vi "Start Function.vi"(8 "error in (no error)":errorcluster, 10 "Launch Functions Message in":refnum<class "Launch Functions Message.lvclass">, 11 "Controller in":refnum<class "Controller.lvclass">) -> (0 "error out":errorcluster, 3 "Controller out":refnum<class "Controller.lvclass">)   [LabVIEW 2016, in "Controller Actor.lvlib" / "Controller.lvclass"]
uses:
  <userlib>/Common Components/Controller/Controller.lvclass
  C:/Program Files (x86)/National Instruments/LabVIEW 2016/vi.lib/ActorFramework/Actor/Actor.lvclass
  <userlib>/Common Components/Controller/Messages/Launch Functions Message/Launch Functions Message.lvclass
  <userlib>/Common Components/Controller/Messages/Launch Functions Message/Launch Functions Message.lvclass/Launch Functions Message.ctl
  <userlib>/Common Components/Hardware/DevInfo/DevInfo.lvclass/DevInfo.ctl
  <userlib>/Common Components/Function Actor/Function.lvclass/Function.ctl
  <vilib>/ActorFramework/Actor/Actor.lvclass/Actor.ctl
  <vilib>/ActorFramework/Message Enqueuer/Message Enqueuer.lvclass/Message Enqueuer.ctl
  <userlib>/Common Components/Function Actor/Accessors/Write Time Function Requested.vi
  <userlib>/Common Components/Function Actor/Write GUID.vi
  <userlib>/Common Components/Function Actor/Accessors/Write Master_.vi
  <userlib>/Common Components/Function Actor/Accessors/Write WS Message Broker Interface Ref.vi
  <userlib>/Common Components/Function Actor/Accessors/Write HWplugin List LUT.vi
  <userlib>/Common Components/Controller/Messages/Launch Functions Message/Read Function Name.vi
  <userlib>/Common Components/Controller/Messages/Launch Functions Message/Read Devices.vi
  <userlib>/Common Components/Controller/Messages/Launch Functions Message/Read Show FP_.vi
  <userlib>/Common Components/Controller/Messages/Launch Functions Message/Read Time Function Requested 2.vi
  <userlib>/Common Components/Controller/Messages/Launch Functions Message/Read Master_.vi
  <vilib>/ActorFramework/Message Enqueuer/Init from Existing Queue.vi
  <userlib>/Common Components/Function Actor/Function.lvclass
  <userlib>/Common Components/Controller/Methods/Print List of Hardware (DevInfo).vi
  <userlib>/Common Components/Function Actor/Properties/Write Array of Hardware 2.vi
  <userlib>/Common Components/Function Actor/Properties/Write Show UI While Running 2.vi
  <userlib>/Common Components/Hardware/DevInfo/DevInfo.lvclass
  <userlib>/Common Components/Hardware/Abstract Hardware/Hardware.lvclass
  <vilib>/ActorFramework/Message Enqueuer/Message Enqueuer.lvclass
  <vilib>/ActorFramework/Actor/Actor.lvclass
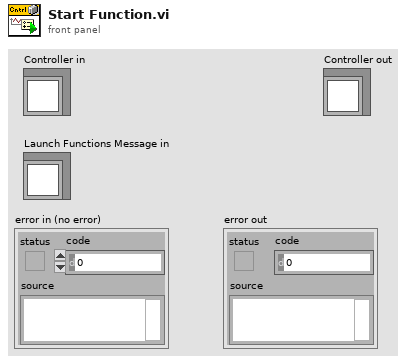
[diagram p1: front panel]
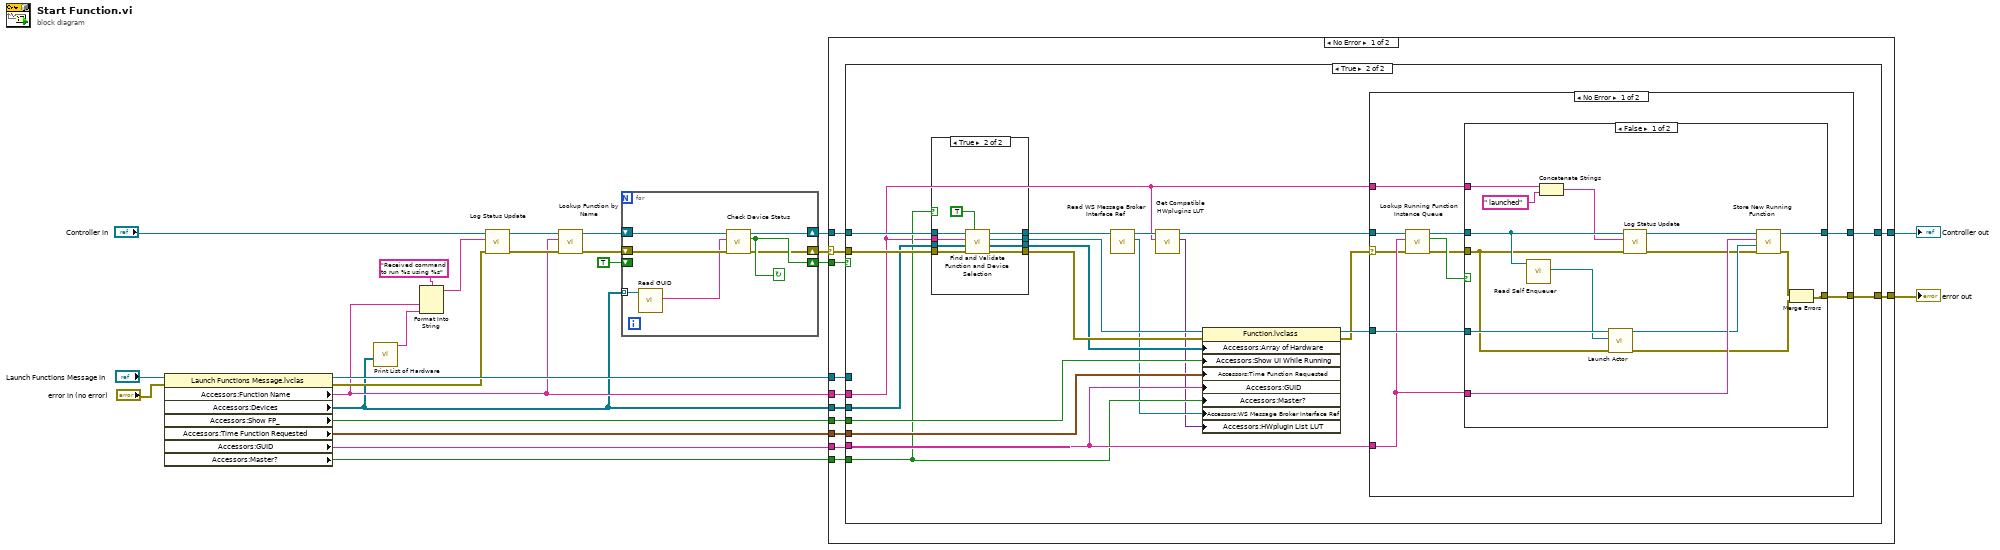
[diagram p0: block diagram]
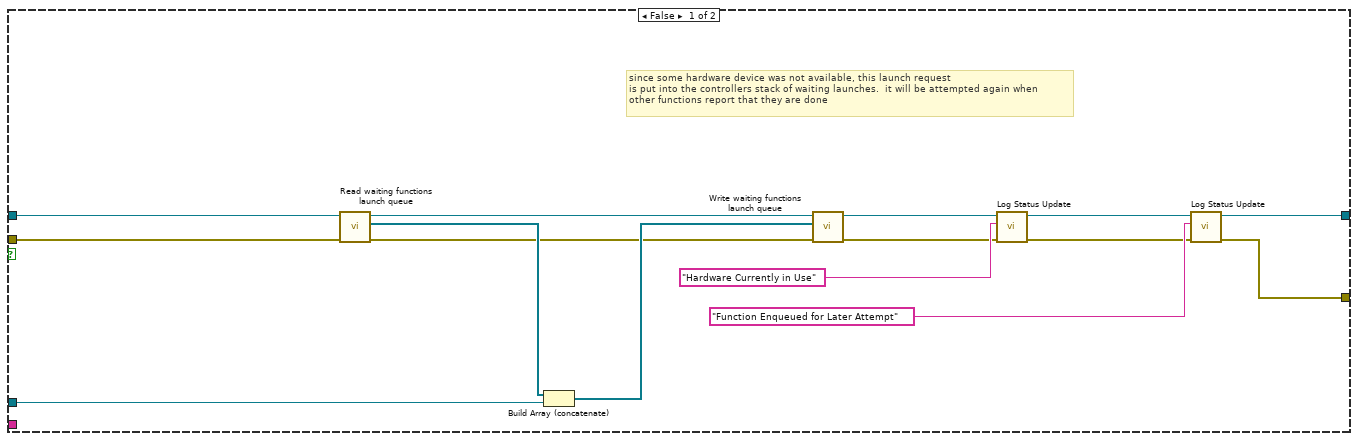
[diagram p2: hidden frame]
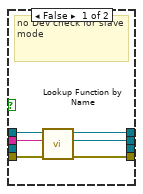
[diagram p3: hidden frame]
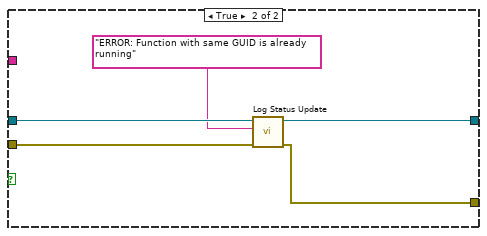
[diagram p4: hidden frame]
diagram:
  n1 = property class="Launch Functions Message.lvclas"(reference="Launch Functions Message in", error in="error in (no error)") -> (reference out=w14:refnum<class "Launch Functions Message.lvclass">, error out=w9:errorcluster, "Accessors:Function Name"=w4:string, "Accessors:Devices"=w3:refnum<class "DevInfo.lvclass">[], "Accessors:Show FP_"=w11:bool, "Accessors:Time Function Requested"=w10:timestamp, "Accessors:GUID"=w13:string, "Accessors:Master?"=w2:bool)
  n2 = call-poly <userlib>:"Print List of Hardware.vi"("Devices"=w3) -> ("String"=w23:string)  [unwired: 10 in]
  n3 = Format Into String(format string="Received command to run %s using %s", w4, w23) -> (resulting string=w22:string)  [unwired: 2 in, 1 out]
  n4 = call-dynamic "Log Status Update.vi"("error in (no error)"=w9, "String"=w22, "Controller in"="Controller in") -> ("error out"=w7:errorcluster, "Controller out"=w8:refnum<class "Controller.lvclass">)  [unwired: 7 in]
  n5 = call <userlib>:"Lookup Function by Name.vi"("error in (no error)"=w7, "Function Name"=w4, "Controller in"=w8) -> ("error out"=w6:errorcluster, "Controller out"=w5:refnum<class "Controller.lvclass">)  [unwired: 5 in, 2 out]
  n6 = for {
    shift-right: [w30] -> w19
    shift-left: w5 -> [w31]
    tunnel: w3 -> [w29] mode=indexing
    shift-right: [w27] -> w18
    shift-left: w6 -> [w26]
    shift-right: [w28] -> w20
    shift-left: TRUE -> [_]
    stop <- w28 continue-if-true
    n7 = call <userlib>:"Read GUID.vi"("DevInfo in"=w29) -> ("GUID"=w25:string)  [unwired: 8 in, 2 out]
    n8 = call <userlib>:"Check Device Status.vi"("error in (no error)"=w26, "Device GUID"=w25, "Controller in"=w31) -> ("error out"=w27:errorcluster, "Available?"=w28:bool, "Controller out"=w30:refnum<class "Controller.lvclass">)  [unwired: 6 in]
  }
  n9 = case shown="No Error" w18 {
    selector: w18 -> [w37 w127]
    tunnel: w20 -> [w43 _]
    tunnel: w19 -> [w42 w126]
    tunnel: [w41 w126] -> w16
    tunnel: w13 -> [w40 _]
    tunnel: [w39 w127] -> w15
    tunnel: w14 -> [w38 _]
    tunnel: w11 -> [w36 _]
    tunnel: w10 -> [w35 _]
    tunnel: w4 -> [w34 _]
    tunnel: w3 -> [w33 _]
    tunnel: w2 -> [w32 _]
    frame No Error {
      n10 = case shown="True" w43 {
        tunnel: [w45 w78] -> w41
        tunnel: w42 -> [w56 w76]
        tunnel: w37 -> [w54 w75]
        tunnel: [w46 w74] -> w39
        tunnel: w40 -> [_ w68]
        tunnel: w38 -> [w44 _]
        tunnel: w36 -> [_ w66]
        tunnel: w35 -> [_ w67]
        tunnel: w34 -> [_ w59]
        tunnel: w33 -> [_ w69]
        tunnel: w32 -> [_ w65]
        frame False {
          # "since some hardware device was not available, this launch request\nis put into the controllers stack of waiting launches.  it will be attempted again when\nother functions report that they are done"
          n11 = call <userlib>:"Read waiting functions launch queue.vi"("error in (no error)"=w54, "Controller in"=w56) -> ("error out"=w53:errorcluster, "stack of waiting fcn requests"=w58:refnum<class "Launch Functions Message.lvclass">[], "Controller out"=w57:refnum<class "Controller.lvclass">)  [unwired: 7 in]
          n12 = Build Array (concatenate)(w58, w44) -> (w55:refnum<class "Launch Functions Message.lvclass">[])
          n13 = call <userlib>:"Write waiting functions launch queue.vi"("error in (no error)"=w53, "stack of waiting fcn requests"=w55, "Controller in"=w57) -> ("error out"=w48:errorcluster, "Controller out"=w49:refnum<class "Controller.lvclass">)  [unwired: 7 in]
          n14 = call-dynamic "Log Status Update.vi"("error in (no error)"=w48, "String"="Hardware Currently in Use", "Controller in"=w49) -> ("error out"=w47:errorcluster, "Controller out"=w50:refnum<class "Controller.lvclass">)  [unwired: 7 in]
          n15 = call-dynamic "Log Status Update.vi"("error in (no error)"=w47, "String"="Function Enqueued for Later Attempt", "Controller in"=w50) -> ("error out"=w46:errorcluster, "Controller out"=w45:refnum<class "Controller.lvclass">)  [unwired: 7 in]
        }
        frame True {
          n16 = case shown="True" w65 {
            tunnel: w76 -> [w84 w93]
            tunnel: w75 -> [w81 w92]
            tunnel: [w83 w91] -> w64
            tunnel: [w80 w90] -> w73
            tunnel: [_ w89] -> w72
            tunnel: [w79 w88] -> w71
            tunnel: w69 -> [_ w87]
            tunnel: w59 -> [w82 w86]
            frame False {
              # "no Dev check for slave mode"
              n17 = call <userlib>:"Lookup Function by Name.vi"("error in (no error)"=w81, "Function Name"=w82, "Controller in"=w84) -> ("error out"=w80:errorcluster, "Function.lvclass"=w79:refnum<class "Function.lvclass">, "Controller out"=w83:refnum<class "Controller.lvclass">)  [unwired: 5 in, 1 out]
            }
            frame True {
              n18 = call <userlib>:"Find and Validate Function and Device Selection.vi"("reserve?"=TRUE, "error in (no error)"=w92, "DevInfos"=w87, "Function Name"=w86, "Controller in"=w93) -> ("error out"=w90:errorcluster, "Hardware Objects"=w89:refnum<class "Hardware.lvclass">[], "Function out"=w88:refnum<class "Function.lvclass">, "Controller out"=w91:refnum<class "Controller.lvclass">)  [unwired: 3 in]
            }
          }
          n19 = call-dynamic "Read WS Message Broker Interface Ref.vi"("Controller in"=w64) -> ("WS Message Broker Interface Ref.lvclass"=w62:refnum<class "WS Message Broker Interface Ref.lvclass">, "Controller out"=w63:refnum<class "Controller.lvclass">)  [unwired: 9 in]
          n20 = call <userlib>:"Get Compatible HWplugins LUT.vi"("Function Name"=w59, "Controller in"=w63) -> ("HWplugin List LUT (HWType -> Array of HWplugin Objs)"=w60:variant, "Controller out"=w61:refnum<class "Controller.lvclass">)  [unwired: 7 in, 1 out]
          n21 = property class="Function.lvclass"(reference=w71, error in=w73, "Accessors:Array of Hardware"=w72, "Accessors:Show UI While Running"=w66, "Accessors:Time Function Requested"=w67, "Accessors:GUID"=w68, "Accessors:Master?"=w65, "Accessors:WS Message Broker Interface Ref"=w62, "Accessors:HWplugin List LUT"=w60) -> (reference out=w77:refnum<class "Function.lvclass">, error out=w70:errorcluster)
          n22 = case shown="No Error" w70 {
            selector: w70 -> [w95 w125]
            tunnel: [w103 w124] -> w78
            tunnel: w77 -> [w99 _]
            tunnel: w61 -> [w98 w124]
            tunnel: w68 -> [w97 _]
            tunnel: [w96 w125] -> w74
            tunnel: w59 -> [w94 _]
            frame No Error {
              n23 = call <userlib>:"Lookup Running Function Instance Queue.vi"("error in (no error)"=w95, "Function Instance Name"=w97, "Controller in"=w98) -> ("error out"=w100:errorcluster, "Found?"=w101:bool, "Controller out"=w102:refnum<class "Controller.lvclass">)  [unwired: 5 in, 1 out]
              n24 = case shown="False" w101 {
                tunnel: [w118 w122] -> w103
                tunnel: w99 -> [w117 _]
                tunnel: w97 -> [w116 _]
                tunnel: w102 -> [w114 w123]
                tunnel: w100 -> [w108 w120]
                tunnel: [w105 w119] -> w96
                tunnel: w94 -> [w104 _]
                frame False {
                  n25 = call <vilib>:"Read Self Enqueuer.vi"("Actor"=w114) -> ("Self Enqueuer"=w113:refnum<class "Message Enqueuer.lvclass">)  [unwired: 10 in]
                  n26 = Concatenate Strings(w104, " launched" ("string")) -> (w110:string)
                  n27 = call <vilib>:"Launch Actor.vi"("error in (no error)"=w108, "Actor-to-Caller Enqueuer"=w113, "Actor"=w117) -> ("error out"=w106:errorcluster, "Caller-To-Actor Enqueuer"=w112:refnum<class "Message Enqueuer.lvclass">)  [unwired: 7 in]
                  n28 = call-dynamic "Log Status Update.vi"("error in (no error)"=w108, "String"=w110, "Controller in"=w114) -> ("error out"=w109:errorcluster, "Controller out"=w111:refnum<class "Controller.lvclass">)  [unwired: 7 in]
                  n29 = call <userlib>:"Store New Running Function.vi"("error in (no error)"=w109, "Caller-To-Actor Enqueuer"=w112, "name"=w116, "Controller in"=w111) -> ("error out"=w107:errorcluster, "Controller out"=w118:refnum<class "Controller.lvclass">)  [unwired: 6 in]
                  n30 = Merge Errors(w107, w106) -> (w105:errorcluster)
                }
                frame True {
                  n31 = call-dynamic "Log Status Update.vi"("error in (no error)"=w120, "String"="ERROR: Function with same GUID is already running", "Controller in"=w123) -> ("error out"=w119:errorcluster, "Controller out"=w122:refnum<class "Controller.lvclass">)  [unwired: 7 in]
                }
              }
            }
            frame Error {
            }
          }
        }
      }
    }
    frame Error {
    }
  }
  "error out" <- w15
  "Controller out" <- w16
